vi "Give Error Source Context.vi"(1 "Context String":string, 7 "error in":errorcluster) -> (8 "Error out with context":errorcluster)   [LabVIEW 2012]
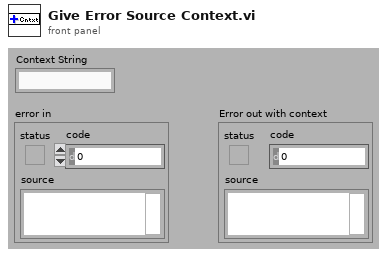
[diagram p1: front panel]
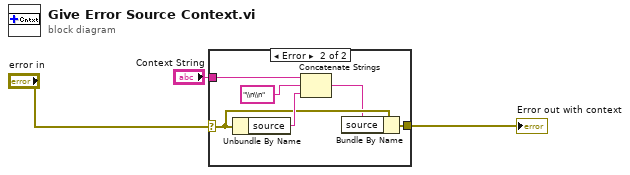
[diagram p0: block diagram]
diagram:
  n1 = case shown="Error" "error in" {
    selector: "error in" -> [w4 w8]
    tunnel: [w4 w9] -> w2
    tunnel: "Context String" -> [_ w6]
    frame No Error {
    }
    frame Error {
      n2 = Unbundle By Name(w8) -> ("source"=w10:string)
      n3 = Concatenate Strings(w6, "\\n\\n" ("string"), w10) -> (w7:string)
      n4 = Bundle By Name(cluster=w8, "source"=w7) -> (w9:errorcluster)
    }
  }
  "Error out with context" <- w2
